vi "G#Object_ParseAttributes.vi"(0 "attributes":variant, 2 "array names (T)":bool=TRUE, 5 "error in (no error)":errorcluster) -> (15 "LabVIEWClassElements":variant[](array[variant]), 16 "array?":bool[](array[boolean]), 17 "attribute name":string[](array[string]), 19 "error out":errorcluster)   [LabVIEW 2020, in "G#Object.lvclass"]
doc: "Parses the attributes cluster and split it into LabVIEW class elements. Clusters and variants are parsed recusively."
uses:
  G#Object.lvclass
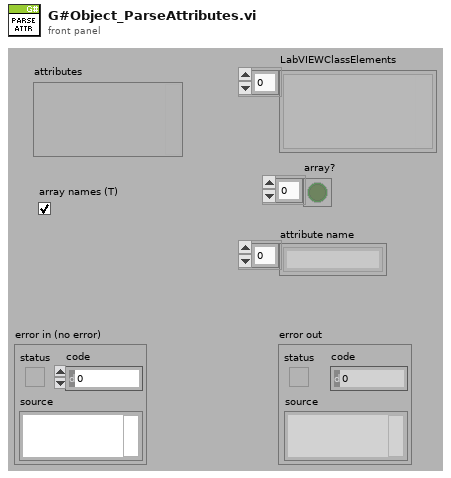
[diagram p1: front panel]
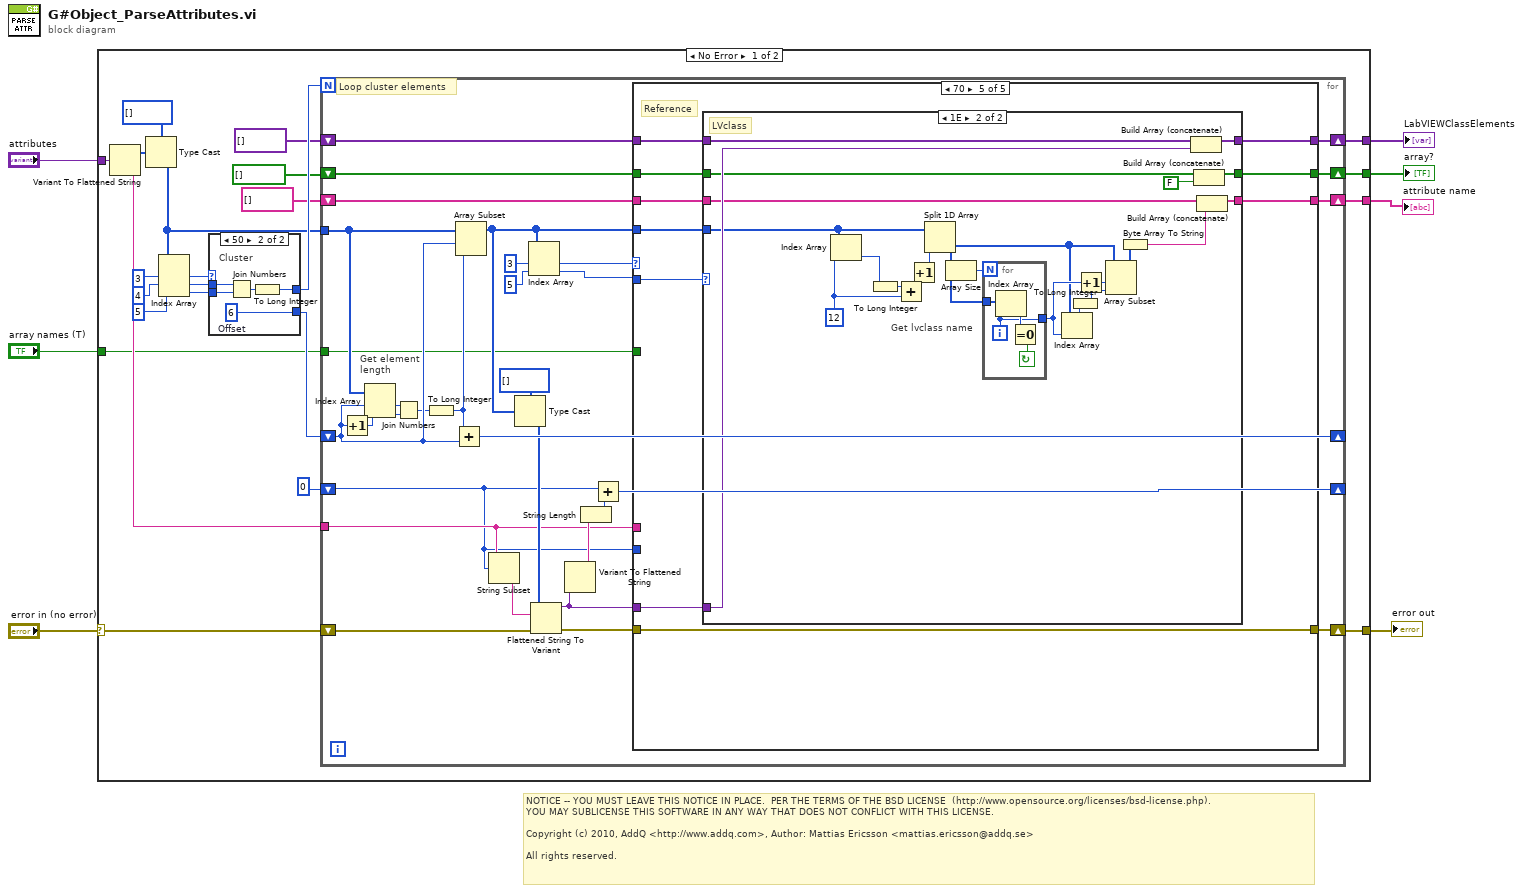
[diagram p0: block diagram]
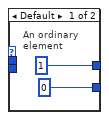
[diagram p2: hidden frame]
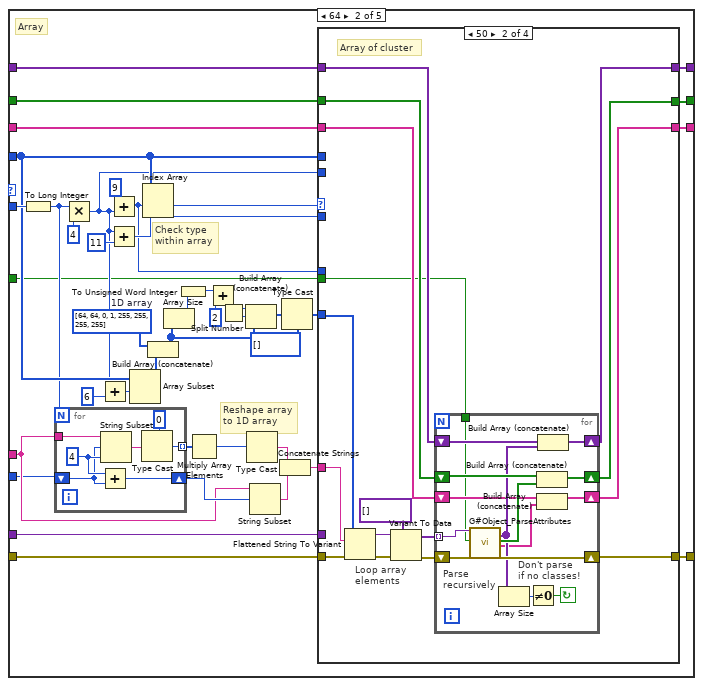
[diagram p4: hidden frame]
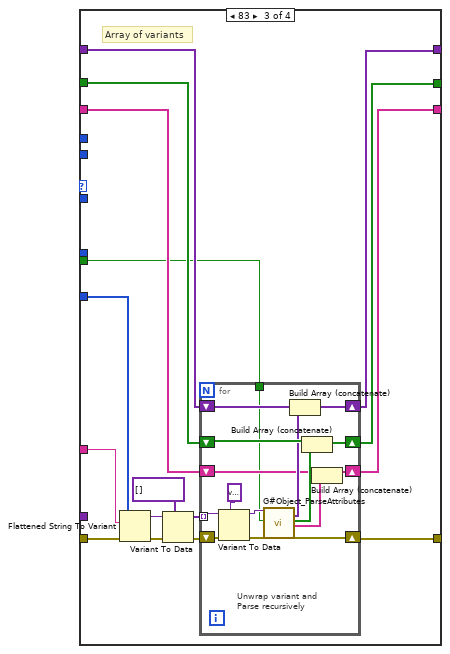
[diagram p6: hidden frame]
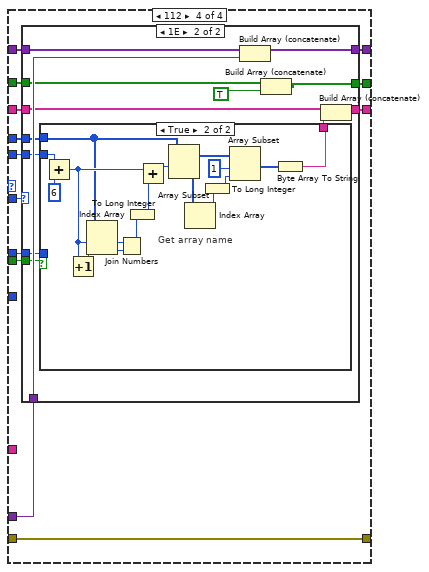
[diagram p7: hidden frame]
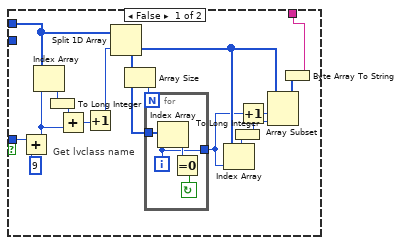
[diagram p9: hidden frame]
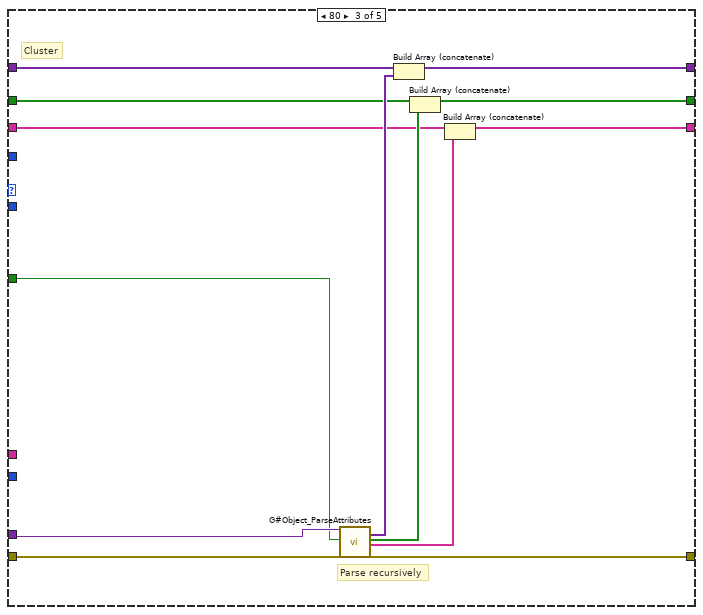
[diagram p10: hidden frame]
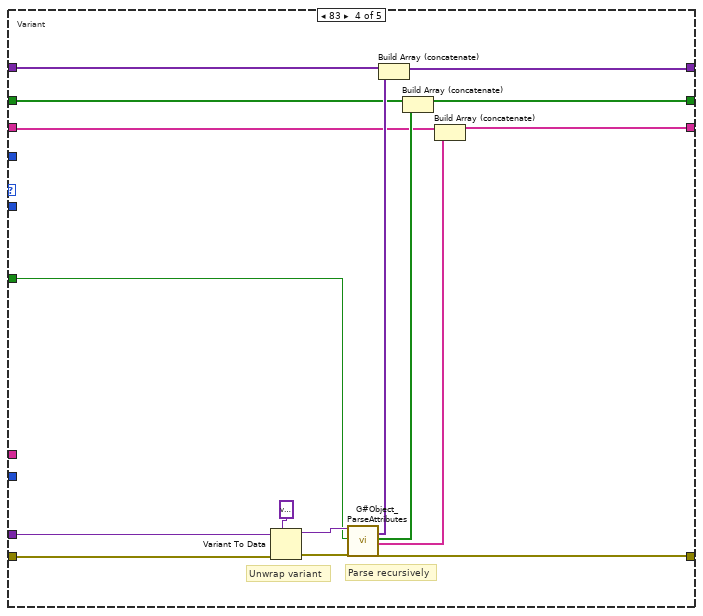
[diagram p11: hidden frame]
diagram:
  # "NOTICE -- YOU MUST LEAVE THIS NOTICE IN PLACE.  PER THE TERMS OF THE BSD LICENSE  (http://www.opensource.org/licenses/bsd-license.php).\nYOU MAY SUBLICENSE THIS SOFTWARE IN ANY WAY THAT DOES NOT CONFLICT WITH THIS LICENSE.\n\nCopyright (c) 2010, AddQ <http://www.addq.com>, Author: Mattias Ericsson <mattias.ericsson@addq.se>\n\nAll rights reserved."
  n1 = case shown="No Error" "error in (no error)" {
    selector: "error in (no error)" -> [w11 w324]
    tunnel: "attributes" -> [w30 _]
    tunnel: [w15 w324] -> w6
    tunnel: [w14 _] -> w5
    tunnel: [w13 _] -> w4
    tunnel: [w9 _] -> w2
    tunnel: "array names (T)" -> [w8 _]
    frame No Error {
      n2 = Variant To Flattened String(Variant=w30) -> (data string=w18:string, 1:w29:i16[])
      n3 = Type Cast(type=u8[] [], x=w29) -> (*(type *) &x=w19:u8[])
      n4 = Index Array(array=w19, index #1=3 ("index"), index #2=4 ("index"), index #3=5 ("index")) -> (element #1=w20:u8, element #2=w22:u8, element #3=w21:u8)
      n5 = case shown="50" w20 {
        tunnel: [1 w36] -> w26
        tunnel: [0 ("Offset") w35] -> w25
        tunnel: w22 -> [_ w34]
        tunnel: w21 -> [_ w33]
        frame Default {
          # "An ordinary\nelement"
        }
        frame 80 {
          w35 = 6  # Offset
          # "Cluster"
          n6 = Join Numbers(hi=w34, lo=w33) -> ((hi.lo)=w37:u16)
          n7 = To Long Integer(number=w37) -> (32bit integer=w36:i32)
        }
      }
      n8 = for {
        N: w26 -> [_]
        tunnel: w19 -> [w69]
        shift-right: [w68] -> _
        shift-left: w25 -> [w64]
        tunnel: w18 -> [w44]
        shift-right: [w53] -> _
        shift-left: 0 ("Offset") -> [w43]
        shift-right: [w49] -> w15
        shift-left: w11 -> [w59]
        shift-right: [w48] -> w14
        shift-left: variant[] [] ("LabVIEWClassElements") -> [w52]
        shift-right: [w47] -> w13
        shift-left: bool[] [] ("Array?") -> [w46]
        shift-right: [w39] -> w9
        shift-left: string[] [] -> [w40]
        tunnel: w8 -> [w38]
        # "Loop cluster elements"
        # "Get element\nlength"
        n9 = Increment(x=w64) -> (x+1=w65:i32)
        n10 = Index Array(array=w69, index #1=w64, index #2=w65) -> (element #1=w66:u8, element #2=w67:u8)
        n11 = Join Numbers(hi=w66, lo=w67) -> ((hi.lo)=w63:u16)
        n12 = To Long Integer(number=w63) -> (32bit integer=w62:i32)
        n13 = Add(x=w62, y=w64) -> (x+y=w68:i32)
        n14 = Array Subset(array=w69, index=w64, length=w62) -> (w45:u8[])
        n15 = String Subset(string=w44, offset (0)=w43) -> (substring=w56:string)  [unwired: 1 in]
        n16 = Type Cast(type=i16[] [] ("type string"), x=w45) -> (*(type *) &x=w57:i16[])
        n17 = Index Array(array=w45, index #1=3 ("index"), index #2=5 ("index")) -> (element #1=w42:u8, element #2=w41:u8)
        n18 = Flattened String To Variant(4:w59, 6:w56, 7:w57) -> (0:w50:errorcluster, 3:w51:variant)
        n19 = Variant To Flattened String(Variant=w51) -> (data string=w55:string)  [unwired: 1 out]
        n20 = String Length(string=w55) -> (length=w54:i32)
        n21 = Add(x=w43, y=w54) -> (x+y=w53:i32)
        n22 = case shown="70" w42 {
          tunnel: w52 -> [w73 w114 w266 w283 w293]
          tunnel: w41 -> [_ w89 _ _ w294]
          tunnel: w51 -> [_ w94 w261 w278 w292]
          tunnel: w50 -> [w72 w116 w268 w279 w288]
          tunnel: [w72 w115 w267 w284 w288] -> w49
          tunnel: [w73 w113 w264 w281 w291] -> w48
          tunnel: [w71 w112 w260 w273 w289] -> w47
          tunnel: w46 -> [w71 w111 w262 w276 w290]
          tunnel: w45 -> [_ w86 _ _ w285]
          tunnel: w44 -> [_ w98 _ _ _]
          tunnel: w43 -> [_ w90 _ _ _]
          tunnel: w40 -> [w70 w88 w258 w272 w287]
          tunnel: [w70 w87 w257 w271 w286] -> w39
          tunnel: w38 -> [_ w82 w256 w269 _]
          frame Default {
          }
          frame 64 {
            w102 = u8[] [64, 64, 0, 1, 255, 255, 255, 255]  # 1D array
            # "Array"
            # "Reshape array\nto 1D array"
            # "Check type\nwithin array"
            n23 = To Long Integer(number=w89) -> (32bit integer=w85:i32)
            n24 = for {
              N: w85 -> [_]
              tunnel: [w121] -> w100 mode=indexing
              shift-right: [w120] -> w99
              shift-left: w90 -> [w117]
              tunnel: w98 -> [w119]
              w118 = 4 ("length")
              n25 = Add(x=w118, y=w117) -> (x+y=w120:i32)
              n26 = String Subset(string=w119, offset (0)=w117, length (rest)=w118) -> (substring=w123:string)
              n27 = Type Cast(type=0, x=w123) -> (*(type *) &x=w121:i32)
            }
            n28 = Multiply(x=w85, y=4) -> (x*y=w84:i32)
            n29 = Add(x=w84, y=6) -> (x+y=w104:i32)
            n30 = Add(x=9, y=w84) -> (x+y=w83:i32)
            n31 = Add(x=w84, y=11) -> (x+y=w108:i32)
            n32 = Array Subset(array=w86, index=w104) -> (w101:u8[])  [unwired: 1 in]
            n33 = Index Array(array=w86, index #1=w83, index #2=w108) -> (element #1=w107:u8, element #2=w106:u8)
            n34 = Build Array (concatenate)(w102, w101) -> (w77:u8[])
            n35 = Array Size(array=w77) -> (size(s)=w80:i32)
            n36 = To Unsigned Word Integer(number=w80) -> (unsigned 16bit integer=w81:u16)
            n37 = Multiply Array Elements(1:w100) -> (0:w97:i32)
            n38 = Add(x=w81, y=u16 2) -> (x+y=w76:u16)
            n39 = Split Number(x=w76) -> (hi(x)=w75:u8, lo(x)=w74:u8)
            n40 = Build Array (concatenate)(w75, w74, w77) -> (w78:u8[])
            n41 = Type Cast(x=w97) -> (*(type *) &x=w96:string)  [unwired: 1 in]
            n42 = String Subset(string=w98, offset (0)=w99) -> (substring=w95:string)  [unwired: 1 in]
            n43 = Concatenate Strings(w96, w95) -> (w93:string)
            n44 = Type Cast(type=i16[] [] ("type string"), x=w78) -> (*(type *) &x=w91:i16[])
            n45 = case shown="50" w107 {
              tunnel: w116 -> [w125 w131 w169 w197]
              tunnel: [w125 w143 w174 w197] -> w115
              tunnel: w114 -> [w127 w142 w173 w202]
              tunnel: w94 -> [_ _ _ w200]
              tunnel: [w127 w140 w171 w201] -> w113
              tunnel: [w126 w139 w170 w199] -> w112
              tunnel: w111 -> [w126 w141 w172 w198]
              tunnel: w106 -> [_ _ _ w203]
              tunnel: w93 -> [_ w136 w167 _]
              tunnel: w91 -> [_ w135 w168 _]
              tunnel: w88 -> [w124 w130 w161 w196]
              tunnel: [w124 w129 w160 w195] -> w87
              tunnel: w86 -> [_ _ _ w194]
              tunnel: w84 -> [_ _ _ w193]
              tunnel: w83 -> [_ _ _ w192]
              tunnel: w82 -> [_ w128 w159 w191]
              frame Default {
              }
              frame 80 {
                # "Loop array\nelements"
                # "Array of cluster"
                n46 = Flattened String To Variant(4:w131, 6:w136, 7:w135) -> (0:w134:errorcluster, 3:w138:variant)
                n47 = Variant To Data(error in=w134, type=variant[] [], Variant=w138) -> (data=w132:variant[], error out=w133:errorcluster)
                n48 = for {
                  tunnel: w132 -> [w149] mode=indexing
                  shift-right: [w155] -> w140
                  shift-left: w142 -> [w156]
                  shift-right: [w154] -> w139
                  shift-left: w141 -> [w153]
                  shift-right: [w157] -> w143
                  shift-left: w133 -> [w158]
                  shift-right: [w146] -> w129
                  shift-left: w130 -> [w148]
                  tunnel: w128 -> [w145]
                  stop <- w144 continue-if-true
                  # "Don't parse\nif no classes!"
                  # "Parse\nrecursively"
                  n49 = call "G#Object_ParseAttributes.vi"("attributes"=w149, "array names (T)"=w145, "error in (no error)"=w158) -> ("LabVIEWClassElements"=w151:variant[], "array?"=w152:bool[], "attribute name"=w147:string[], "error out"=w157:errorcluster)  [unwired: 13 in]
                  n50 = Array Size(array=w151) -> (size(s)=w150:i32)
                  n51 = Not Equal To 0?(x=w150) -> (x != 0?=w144:bool)
                  n52 = Build Array (concatenate)(w153, w152) -> (w154:bool[])
                  n53 = Build Array (concatenate)(w148, w147) -> (w146:string[])
                  n54 = Build Array (concatenate)(w156, w151) -> (w155:variant[])
                }
              }
              frame 83 {
                # "Array of variants"
                n55 = Flattened String To Variant(4:w169, 6:w167, 7:w168) -> (0:w166:errorcluster, 3:w165:variant)
                n56 = Variant To Data(error in=w166, type=variant[] [], Variant=w165) -> (data=w162:variant[], error out=w164:errorcluster)
                n57 = for {
                  tunnel: w162 -> [w182] mode=indexing
                  shift-right: [w188] -> w171
                  shift-left: w173 -> [w189]
                  shift-right: [w179] -> w170
                  shift-left: w172 -> [w187]
                  shift-right: [w190] -> w174
                  shift-left: w164 -> [w184]
                  shift-right: [w176] -> w160
                  shift-left: w161 -> [w178]
                  tunnel: w159 -> [w175]
                  # "Unwrap variant and\nParse recursively"
                  n58 = Variant To Data(error in=w184, type=variant, Variant=w182) -> (data=w180:variant, error out=w183:errorcluster)
                  n59 = call "G#Object_ParseAttributes.vi"("attributes"=w180, "array names (T)"=w175, "error in (no error)"=w183) -> ("LabVIEWClassElements"=w181:variant[], "array?"=w186:bool[], "attribute name"=w177:string[], "error out"=w190:errorcluster)  [unwired: 13 in]
                  n60 = Build Array (concatenate)(w189, w181) -> (w188:variant[])
                  n61 = Build Array (concatenate)(w187, w186) -> (w179:bool[])
                  n62 = Build Array (concatenate)(w178, w177) -> (w176:string[])
                }
              }
              frame 112 {
                n63 = case shown="1E" w203 {
                  tunnel: w202 -> [w206 w219]
                  tunnel: [w206 w218] -> w201
                  tunnel: w200 -> [_ w217]
                  tunnel: [w205 w213] -> w199
                  tunnel: w198 -> [w205 w216]
                  tunnel: w196 -> [w204 w211]
                  tunnel: [w204 w212] -> w195
                  tunnel: w194 -> [_ w214]
                  tunnel: w193 -> [_ w209]
                  tunnel: w192 -> [_ w208]
                  tunnel: w191 -> [_ w207]
                  frame Default {
                  }
                  frame 30 {
                    n64 = case shown="True" w207 {
                      tunnel: w214 -> [w223 w243]
                      tunnel: [w224 w242] -> w210
                      tunnel: w209 -> [_ w240]
                      tunnel: w208 -> [w220 _]
                      frame False {
                        # "Get lvclass name"
                        n65 = Add(x=w220, y=9 ("index")) -> (x+y=w221:i32)
                        n66 = Index Array(array=w223, index=w221) -> (element=w235:u8)
                        n67 = To Long Integer(number=w235) -> (32bit integer=w231:i32)
                        n68 = Add(x=w231, y=w221) -> (x+y=w233:i32)
                        n69 = Increment(x=w233) -> (x+1=w232:i32)
                        n70 = Split 1D Array(array=w223, index=w232) -> (second subarray=w230:u8[])  [unwired: 1 out]
                        n71 = Array Size(array=w230) -> (size(s)=w234:i32)
                        n72 = for {
                          N: w234 -> [_]
                          tunnel: w230 -> [w239]
                          tunnel: [w236] -> w229
                          i -> [w236]
                          stop <- w237 continue-if-true
                          n73 = Index Array(array=w239, index=w236) -> (element=w238:u8)
                          n74 = Equal To 0?(x=w238) -> (x = 0?=w237:bool)
                        }
                        n75 = Index Array(array=w230, index=w229) -> (element=w228:u8)
                        n76 = To Long Integer(number=w228) -> (32bit integer=w227:i32)
                        n77 = Increment(x=w229) -> (x+1=w225:i32)
                        n78 = Array Subset(array=w230, index=w225, length=w227) -> (w226:u8[])
                        n79 = Byte Array To String(unsigned byte array=w226) -> (string=w224:string)
                      }
                      frame True {
                        # "Get array name"
                        n80 = Add(x=w240, y=6 ("x")) -> (x+y=w253:i32)
                        n81 = Increment(x=w253) -> (x+1=w245:i32)
                        n82 = Index Array(array=w243, index #1=w253, index #2=w245) -> (element #1=w246:u8, element #2=w247:u8)
                        n83 = Join Numbers(hi=w246, lo=w247) -> ((hi.lo)=w248:u16)
                        n84 = To Long Integer(number=w248) -> (32bit integer=w254:i32)
                        n85 = Add(x=w253, y=w254) -> (x+y=w244:i32)
                        n86 = Array Subset(array=w243, index=w244) -> (w249:u8[])  [unwired: 1 in]
                        n87 = Index Array(array=w249) -> (element=w250:u8)  [unwired: 1 in]
                        n88 = To Long Integer(number=w250) -> (32bit integer=w255:i32)
                        n89 = Array Subset(array=w249, index=1, length=w255) -> (w252:u8[])
                        n90 = Byte Array To String(unsigned byte array=w252) -> (string=w242:string)
                      }
                    }
                    n91 = Build Array (concatenate)(w219, w217) -> (w218:variant[])
                    n92 = Build Array (concatenate)(w216, TRUE) -> (w213:bool[])
                    n93 = Build Array (concatenate)(w211, w210) -> (w212:string[])
                  }
                }
              }
            }
          }
          frame 80 {
            # "Parse recursively"
            # "Cluster"
            n94 = call "G#Object_ParseAttributes.vi"("attributes"=w261, "array names (T)"=w256, "error in (no error)"=w268) -> ("LabVIEWClassElements"=w265:variant[], "array?"=w263:bool[], "attribute name"=w259:string[], "error out"=w267:errorcluster)  [unwired: 13 in]
            n95 = Build Array (concatenate)(w266, w265) -> (w264:variant[])
            n96 = Build Array (concatenate)(w262, w263) -> (w260:bool[])
            n97 = Build Array (concatenate)(w258, w259) -> (w257:string[])
          }
          frame 83 {
            # "Unwrap variant"
            # "Parse recursively"
            # "Variant"
            n98 = Variant To Data(error in=w279, type=variant, Variant=w278) -> (data=w274:variant, error out=w277:errorcluster)
            n99 = call "G#Object_ParseAttributes.vi"("attributes"=w274, "array names (T)"=w269, "error in (no error)"=w277) -> ("LabVIEWClassElements"=w282:variant[], "array?"=w275:bool[], "attribute name"=w270:string[], "error out"=w284:errorcluster)  [unwired: 13 in]
            n100 = Build Array (concatenate)(w283, w282) -> (w281:variant[])
            n101 = Build Array (concatenate)(w276, w275) -> (w273:bool[])
            n102 = Build Array (concatenate)(w272, w270) -> (w271:string[])
          }
          frame 112 {
            # "Reference"
            n103 = case shown="1E" w294 {
              tunnel: w293 -> [w297 w319]
              tunnel: w292 -> [_ w318]
              tunnel: [w297 w317] -> w291
              tunnel: w290 -> [w296 w316]
              tunnel: [w296 w315] -> w289
              tunnel: w287 -> [w295 w313]
              tunnel: [w295 w312] -> w286
              tunnel: w285 -> [_ w299]
              frame Default {
              }
              frame 30 {
                w301 = 12 ("index")
                # "Get lvclass name"
                # "LVclass"
                n104 = Index Array(array=w299, index=w301) -> (element=w300:u8)
                n105 = To Long Integer(number=w300) -> (32bit integer=w305:i32)
                n106 = Add(x=w305, y=w301) -> (x+y=w303:i32)
                n107 = Increment(x=w303) -> (x+1=w304:i32)
                n108 = Split 1D Array(array=w299, index=w304) -> (second subarray=w306:u8[])  [unwired: 1 out]
                n109 = Array Size(array=w306) -> (size(s)=w302:i32)
                n110 = for {
                  N: w302 -> [_]
                  tunnel: w306 -> [w323]
                  tunnel: [w320] -> w307
                  i -> [w320]
                  stop <- w321 continue-if-true
                  n111 = Index Array(array=w323, index=w320) -> (element=w322:u8)
                  n112 = Equal To 0?(x=w322) -> (x = 0?=w321:bool)
                }
                n113 = Index Array(array=w306, index=w307) -> (element=w308:u8)
                n114 = To Long Integer(number=w308) -> (32bit integer=w309:i32)
                n115 = Increment(x=w307) -> (x+1=w311:i32)
                n116 = Array Subset(array=w306, index=w311, length=w309) -> (w310:u8[])
                n117 = Byte Array To String(unsigned byte array=w310) -> (string=w298:string)
                n118 = Build Array (concatenate)(w319, w318) -> (w317:variant[])
                n119 = Build Array (concatenate)(w316, FALSE ("Array")) -> (w315:bool[])
                n120 = Build Array (concatenate)(w313, w298) -> (w312:string[])
              }
            }
          }
        }
      }
    }
    frame Error {
    }
  }
  "error out" <- w6
  "LabVIEWClassElements" <- w5
  "array?" <- w4
  "attribute name" <- w2
